vi "sub_clustering.vi"(11 "2d data":cluster{"X":dbl, "Y":dbl}[](graph)) -> (3 "clustering":cluster{"X":dbl, "Y":dbl}[](graph))   [LabVIEW 2019]
panel:
  out "XY Graph":cluster{"X":dbl, "Y":dbl}[](graph)
  in  "stop":bool
  in  "index":i32
  out "size(s)":i32
  out "sorted array":T1(array[cluster])
  in  "limit_ptn":u8
  in  "limit_len":dbl
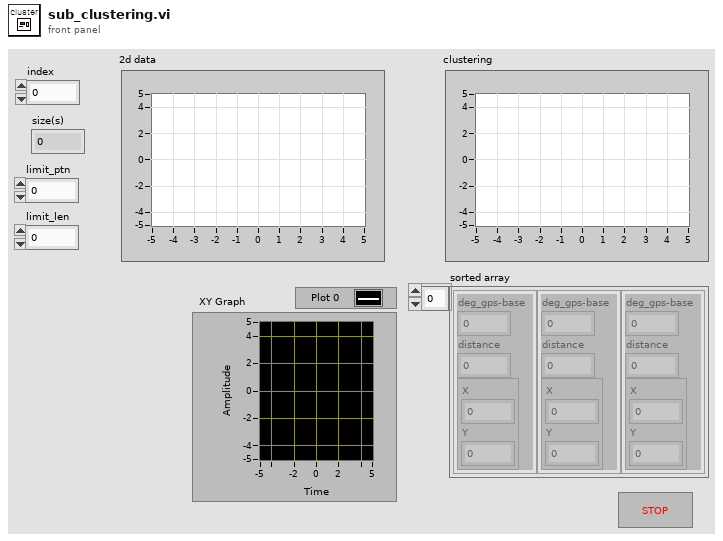
[diagram p1: front panel]
types:
  T1 = cluster{"deg_gps-base":dbl, "distance":dbl, cluster{"X":dbl, "Y":dbl}}[]
  T2 = cluster{"theta":dbl, "r":dbl, "xy":cluster{"X":dbl, "Y":dbl}}
  T3 = cluster{"theta":dbl, "r":dbl, "xy":cluster{"X":dbl, "Y":dbl}}[]
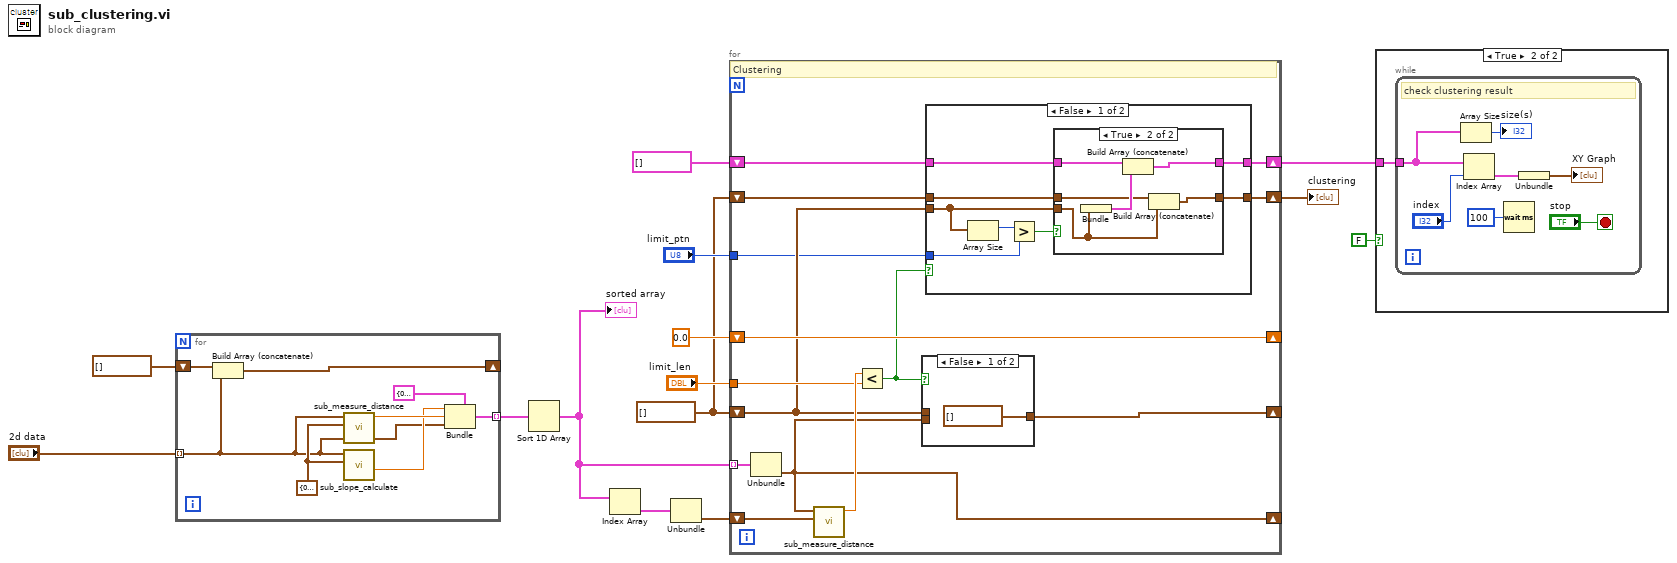
[diagram p0: block diagram]
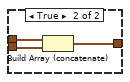
[diagram p5: hidden frame]
diagram:
  w3 = cluster{"x":dbl, "y":dbl}[] [] ("Array")
  n1 = for {
    tunnel: "2d data" -> [w16] mode=indexing
    shift-right: [w21] -> _
    shift-left: cluster{"X":dbl, "Y":dbl}[] [] -> [w22]
    tunnel: [w19] -> w8 mode=indexing
    w20 = cluster{"x":dbl, "y":dbl} {"x"=0.0, "y"=0.0} ("pt 2")
    n2 = Build Array (concatenate)(w22, w16) -> (w21:cluster{"X":dbl, "Y":dbl}[])
    n3 = call "sub_measure_distance.vi"("pt 2"=w20, "pt 1"=w16) -> ("distance"=w18:dbl)  [unwired: 9 in]
    n4 = call "sub_slope_calculate.vi"("point n+1"=w20, "point n"=w16) -> ("deg_gps-base"=w17:dbl)  [unwired: 7 in, 2 out]
    n5 = Bundle(cluster=T2 {"theta"=0.0, "r"=0.0, "xy"={"X"=0.0, "Y"=0.0}}, "theta"=w17, "r"=w18, "xy"=w16) -> (w19:T2)
  }
  n6 = Sort 1D Array(array=w8) -> (sorted array=w6:T3)
  "sorted array" <- w6
  n7 = Index Array(array=w6) -> (element=w5:T2)  [unwired: 1 in]
  n8 = Unbundle(w5) -> ("xy"=w4:cluster{"X":dbl, "Y":dbl})  [unwired: 2 out]
  n9 = for {
    shift-right: [w29] -> _
    shift-left: w4 -> [w36]
    shift-right: [w33] -> w10
    shift-left: cluster{"Array":cluster{"x":dbl, "y":dbl}[]}[] [] ("Array") -> [w34]
    shift-right: [w35] -> _
    shift-left: 0.0 -> [w35]
    tunnel: "limit_len" -> [w31]
    tunnel: "limit_ptn" -> [w25]
    shift-right: [w27] -> _
    shift-left: w3 -> [w26]
    tunnel: w6 -> [w30] mode=indexing
    shift-right: [w23] -> w1
    shift-left: w3 -> [w24]
    # "Clustering"
    n10 = Unbundle(w30) -> ("xy"=w29:cluster{"X":dbl, "Y":dbl})  [unwired: 2 out]
    n11 = call "sub_measure_distance.vi"("pt 2"=w36, "pt 1"=w29) -> ("distance"=w32:dbl)  [unwired: 9 in]
    n12 = Less?(x=w32, y=w31) -> (x < y?=w28:bool)
    n13 = case shown="False" w28 {
      tunnel: w26 -> [_ w58]
      tunnel: w29 -> [_ w57]
      tunnel: [cluster{"x":dbl, "y":dbl}[] [] w56] -> w27
      frame False {
      }
      frame True {
        n14 = Build Array (concatenate)(w58, w57) -> (w56:cluster{"X":dbl, "Y":dbl}[])
      }
    }
    n15 = case shown="False" w28 {
      tunnel: w26 -> [w42 _]
      tunnel: w34 -> [w44 w54]
      tunnel: [w43 w54] -> w33
      tunnel: w25 -> [w39 _]
      tunnel: w24 -> [w38 w53]
      tunnel: [w37 w53] -> w23
      frame False {
        n16 = Array Size(array=w42) -> (size(s)=w41:i32)
        n17 = Greater?(x=w41, y=w39) -> (0:w40:bool)
        n18 = case shown="True" w40 {
          tunnel: w44 -> [w46 w51]
          tunnel: [w46 w50] -> w43
          tunnel: w42 -> [_ w49]
          tunnel: w38 -> [w45 w48]
          tunnel: [w45 w47] -> w37
          frame False {
          }
          frame True {
            n19 = Bundle("Array"=w49) -> (w52:cluster{"Array":cluster{"x":dbl, "y":dbl}[]})  [unwired: 1 in]
            n20 = Build Array (concatenate)(w51, w52) -> (w50:cluster{"Array":cluster{"x":dbl, "y":dbl}[]}[])
            n21 = Build Array (concatenate)(w48, w49) -> (w47:cluster{"x":dbl, "y":dbl}[])
          }
        }
      }
      frame True {
      }
    }
  }
  "clustering" <- w1
  n22 = case shown="True" FALSE {
    tunnel: w10 -> [_ w59]
    frame False {
    }
    frame True {
      n23 = while {
        tunnel: w59 -> [w61]
        stop <- "stop" stop-if-true
        # "check clustering result"
        n24 = Array Size(array=w61) -> (size(s)=→"size(s)":i32)
        n25 = Index Array(array=w61, index="index") -> (element=w63:cluster{"Array":cluster{"x":dbl, "y":dbl}[]})
        n26 = Wait (ms)(milliseconds to wait=u32 100) -> ()  [unwired: 1 out]
        n27 = Unbundle(w63) -> ("Array"=→"XY Graph":cluster{"x":dbl, "y":dbl}[])
      }
    }
  }
